vi "Convert to RPM (analog).vi"(2 "tacho info":T1={"threshold [V]"=1.0, "pulse width (2)"=2, "avg on n pulses (2)"=2, "pulse/revolution (1)"=1} {"pulse/revolution (1)" min=1 step=1; "avg on n pulses (2)" min=2 step=1; "pulse width (2)" min=1; "threshold [V]" format="%.2f"}, 3 "sampling frequency [Hz]":dbl=10000.0 format="%.2f", 4 "tacho signal [V]":dbl[](array[numeric]) format="%.2f") -> (0 "rpm vs. indices":cluster{"indices":dbl[], "speed [rpm]":dbl[]} {"speed [rpm]" format="%.2f"; "indices" format="%.2f"}, 1 "rpm vs. time":cluster{"time [s]":dbl[], "speed [rpm]":dbl[]} {"speed [rpm]" format="%.2f"; "time [s]" format="%.2f"})   [LabVIEW 2017]
doc: "Converts the signal acquired by a tachometer (pulse train) into a rotational speed, expressed in revolutions per minute (rpm), versus time curve.\nThe tacho info cluster specifies the characteristics of the pulses generated by the tachometer (threshold and pulse width), the number of pulses per revolution, and the number of pulses used to compute the rotational speed.\nThis VI returns the rotational speed as a function of indices, which allows you to perform additional analysis at any specific rotational speed."
uses:
  <vilib>/Analysis/NI_AALPro.lvlib
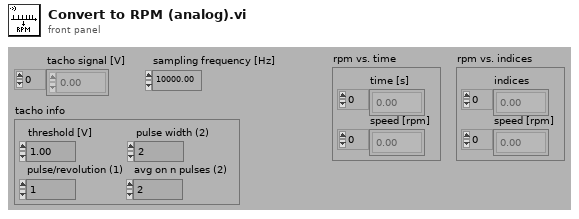
[diagram p1: front panel]
types:
  T1 = cluster{"threshold [V]":dbl, "pulse width (2)":i32, "avg on n pulses (2)":i32, "pulse/revolution (1)":i32}
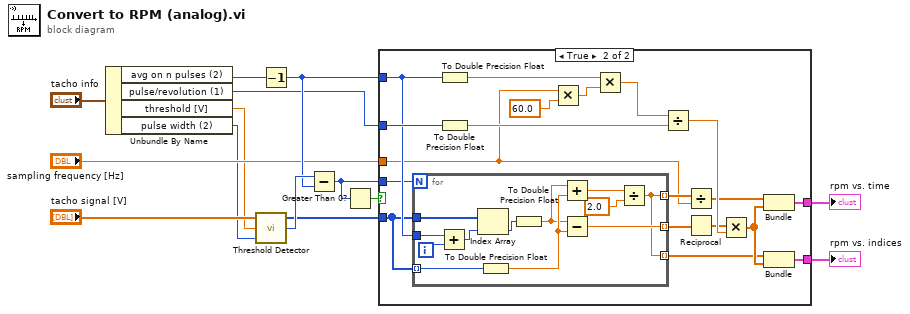
[diagram p0: block diagram]
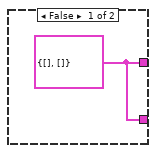
[diagram p2: hidden frame]
diagram:
  n1 = Unbundle By Name("tacho info") -> ("avg on n pulses (2)"=w2:i32, "pulse/revolution (1)"=w1:i32, "threshold [V]"=w4:dbl, "pulse width (2)"=w3:i32)
  n2 = call <vilib>:"Threshold Detector.vi"("width"=w3, "threshold"=w4, "X"="tacho signal [V]") -> ("count"=w14:i32, "Indices"=w12:i32[])  [unwired: 1 out]
  n3 = Decrement(x=w2) -> (x-1=w13:i32)
  n4 = Subtract(x=w14, y=w13) -> (x-y=w8:i32)
  n5 = Greater Than 0?(x=w8) -> (x > 0?=w7:bool)
  n6 = case shown="True" w7 {
    tunnel: w8 -> [_ w20]
    tunnel: w1 -> [_ w33]
    tunnel: w13 -> [_ w29]
    tunnel: w12 -> [_ w27]
    tunnel: "sampling frequency [Hz]" -> [_ w19]
    tunnel: [w15 w21] -> w9
    tunnel: [w15 w18] -> w6
    frame False {
      w15 = cluster{dbl[], dbl[]} {[], []}
    }
    frame True {
      n7 = for {
        N: w20 -> [_]
        tunnel: w27 -> [w46]
        tunnel: [w45] -> w32 mode=indexing
        tunnel: w27 -> [w41] mode=indexing
        tunnel: w29 -> [w43]
        tunnel: [w35] -> w26 mode=indexing
        tunnel: [w35] -> w16 mode=indexing
        i -> [w42]
        n8 = Add(x=w43, y=w42) -> (x+y=w44:i32)
        n9 = Index Array(array=w46, index=w44) -> (element=w40:i32)
        n10 = To Double Precision Float(number=w41) -> (double precision float=w38:dbl)
        n11 = To Double Precision Float(number=w40) -> (double precision float=w37:dbl)
        n12 = Add(x=w37, y=w38) -> (x+y=w39:dbl)
        n13 = Subtract(x=w37, y=w38) -> (x-y=w45:dbl)
        n14 = Divide(x=w39, y=2.0) -> (x/y=w35:dbl)
      }
      n15 = To Double Precision Float(number=w29) -> (double precision float=w23:dbl)
      n16 = To Double Precision Float(number=w33) -> (double precision float=w22:dbl)
      n17 = Multiply(x=w19, y=60.0) -> (x*y=w30:dbl)
      n18 = Multiply(x=w23, y=w30) -> (x*y=w28:dbl)
      n19 = Divide(x=w28, y=w22) -> (x/y=w34:dbl)
      n20 = Divide(x=w26, y=w19) -> (x/y=w25:dbl[])
      n21 = Reciprocal(x=w32) -> (1/x=w24:dbl[])
      n22 = Multiply(x=w24, y=w34) -> (x*y=w17:dbl[])
      n23 = Bundle(w25, w17) -> (w21:cluster{dbl[], dbl[]})  [unwired: 1 in]
      n24 = Bundle(w16, w17) -> (w18:cluster{dbl[], dbl[]})  [unwired: 1 in]
    }
  }
  "rpm vs. time" <- w9
  "rpm vs. indices" <- w6
